vi "Main.vi"(7 "sweep rate, /min":dbl=0.2, 8 "sweep to:":dbl=4.0, 9 "sweep":T8(radio)=enum."2636a_smub") -> ()   [LabVIEW 2021] (continued)
              n2485 = property on="XY Graph" class="XYGraph (strict)"(error in=w3491, "YScale.NameLbl.Text"=w3485) -> ()  [unwired: 1 in, 2 out]
            }
            frame #1 {
              n2486 = local read "Xaxis"() -> (w3508:u16)
              n2487 = property on="Yright" class="Ring (strict)"() -> ("Value"=w3502:u16)  [unwired: 2 in, 2 out]
              n2488 = property on="Yright" class="Ring (strict)"() -> ("RingText.Text"=w3501:string)  [unwired: 2 in, 2 out]
              n2489 = property on="Xaxis" class="Ring (strict)"() -> ("RingText.Text"=w3507:string)  [unwired: 2 in, 2 out]
              n2490 = property on="Yaxis" class="Ring (strict)"() -> ("RingText.Text"=w3506:string)  [unwired: 2 in, 2 out]
              n2491 = local read "Yaxis"() -> (w3509:u16)
              n2492 = case shown="\"0\", Default" w3501 {
                tunnel: [w3514 w3521] -> w3499
                tunnel: w3502 -> [_ w3520]
                tunnel: w3503 -> [w3515 w3519]
                tunnel: [w3513 errorcluster {"status"=FALSE, "code"=0, "source"=""} ("error out")] -> _
                frame "formula" {
                  n2493 = local read "formula_variables"() -> (w3516:string[])
                  n2494 = Transpose 2D Array(2D array=w3515) -> (transposed array=w3517:dbl[][])
                  n2495 = property on="Y_right_formula" class="Str"() -> ("Value"=w3512:string)  [unwired: 2 in, 2 out]
                  n2496 = call <vilib>:"Eval Multi-Variable Array.vi"("Variables"=w3516, "X Values"=w3517, "formula"=w3512) -> ("error out"=w3513:errorcluster, "Y Values"=w3514:dbl[])  [unwired: 1 in]
                }
                frame "0", Default {
                  n2497 = Index Array(array=w3519, index (col)=w3520) -> (element=w3521:dbl[])  [unwired: 1 in]
                }
              }
              n2498 = case shown="\"formula\"" w3507 {
                tunnel: [w3532 w3537] -> w3511
                tunnel: w3508 -> [w3535 _]
                tunnel: w3503 -> [w3534 w3541]
                tunnel: [errorcluster {"status"=FALSE, "code"=0, "source"=""} ("error out") w3538] -> w3505
                tunnel: [w3532 w3537] -> w3500
                frame "0", Default {
                  n2499 = Index Array(array=w3534, index (col)=w3535) -> (element=w3532:dbl[])  [unwired: 1 in]
                }
                frame "formula" {
                  n2500 = local read "formula_variables"() -> (w3540:string[])
                  n2501 = Transpose 2D Array(2D array=w3541) -> (transposed array=w3539:dbl[][])
                  n2502 = property on="X_axis_formula" class="Str"() -> ("Value"=w3536:string)  [unwired: 2 in, 2 out]
                  n2503 = call <vilib>:"Eval Multi-Variable Array.vi"("Variables"=w3540, "X Values"=w3539, "formula"=w3536) -> ("error out"=w3538:errorcluster, "Y Values"=w3537:dbl[])  [unwired: 1 in]
                }
              }
              n2504 = case shown="\"formula\"" w3506 {
                tunnel: [w3524 w3531] -> w3510
                tunnel: w3509 -> [_ w3530]
                tunnel: w3503 -> [w3525 w3529]
                tunnel: [w3523 errorcluster {"status"=FALSE, "code"=0, "source"=""} ("error out")] -> w3504
                frame "formula" {
                  n2505 = local read "formula_variables"() -> (w3526:string[])
                  n2506 = Transpose 2D Array(2D array=w3525) -> (transposed array=w3527:dbl[][])
                  n2507 = property on="Y_left_formula" class="Str"() -> ("Value"=w3522:string)  [unwired: 2 in, 2 out]
                  n2508 = call <vilib>:"Eval Multi-Variable Array.vi"("Variables"=w3526, "X Values"=w3527, "formula"=w3522) -> ("error out"=w3523:errorcluster, "Y Values"=w3524:dbl[])  [unwired: 1 in]
                }
                frame "0", Default {
                  n2509 = Index Array(array=w3529, index (col)=w3530) -> (element=w3531:dbl[])  [unwired: 1 in]
                }
              }
              n2510 = Bundle("Y Values"=w3511, "Y Values"=w3510) -> (w3498:cluster{"Y Values":dbl[], "Y Values":dbl[]})  [unwired: 1 in]
              n2511 = Bundle("Y Values"=w3500, "Y Values"=w3499) -> (w3497:cluster{"Y Values":dbl[], "Y Values":dbl[]})  [unwired: 1 in]
              n2512 = Build Array(w3498, w3497) -> (w3496:cluster{"Y Values":dbl[], "Y Values":dbl[]}[])
              n2513 = property on="XY Graph" class="XYGraph (strict)"("Value"=w3496) -> ()  [unwired: 2 in, 2 out]
            }
            frame #2 {
              # "show if formula \nis wrong"
              n2514 = property on="Yaxis" class="Ring (strict)"() -> ("RingText.Text"=w3547:string)  [unwired: 2 in, 2 out]
              n2515 = property on="XY Graph" class="XYGraph (strict)"("Active Plot"=u32 0, "Plot.Plot Name"=w3547) -> (error out=w3548:errorcluster)  [unwired: 2 in, 1 out]
              n2516 = property on="Yright" class="Ring (strict)"() -> ("RingText.Text"=w3545:string)  [unwired: 2 in, 2 out]
              n2517 = property on="XY Graph" class="XYGraph (strict)"(error in=w3548, "Active Plot"=u32 1, "Plot.Plot Name"=w3545) -> ()  [unwired: 1 in, 2 out]
              n2518 = Unbundle By Name(w3551) -> ("status"=w3544:bool)
              n2519 = Unbundle By Name(w3550) -> ("status"=w3543:bool)
              n2520 = Unbundle By Name(w3550) -> ("status"=w3542:bool)
              n2521 = property on="status 3" class="Bool (strict)"("Value"=w3542) -> ()  [unwired: 2 in, 2 out]
              n2522 = property on="status 2" class="Bool (strict)"("Value"=w3544) -> ()  [unwired: 2 in, 2 out]
              n2523 = property on="status" class="Bool (strict)"("Value"=w3543) -> ()  [unwired: 2 in, 2 out]
            }
          }
          n2524 = stacked-sequence "set next value in the sweep" {
            tunnel: w2536 -> [w3354 _]
            tunnel: [w3354 _] -> w2535
            tunnel: w2533 -> [_ w3475]
            tunnel: w2528 -> [w3357 _]
            frame #0 {
              n2525 = local read "sweep"() -> (w3360:T8)
              n2526 = property on="Sweep Channel" class="DigNum (strict)"("Value"=w3354) -> ()  [unwired: 2 in, 2 out]
              n2527 = property on="sweep value" class="DigNum (strict)"("Value"=w3354) -> ()  [unwired: 2 in, 2 out]
              n2528 = case shown="\"AuxOut0\"" w3360 {
                tunnel: w3354 -> [w3373 w3381 w3387 w3396 w3418 _ w3420 w3443 w3467 w3470]
                tunnel: w3357 -> [_ _ _ w3394 _ _ _ _ _ _]
                frame "2400_1" {
                  # "sweep voltage on 2400 1"
                  n2529 = local read "2400 1 addr"() -> (w3375:u8)
                  n2530 = Number To Fractional String(number=w3373) -> (F-format string=w3379:string)  [unwired: 3 in]
                  n2531 = Concatenate Strings(":INIT:IMM; :SOUR:VOLT:LEV:IMM:AMPL " ("data"), w3379) -> (w3377:string)
                  n2532 = Number To Decimal String(number=w3375) -> (decimal integer string=w3374:string)  [unwired: 1 in]
                  n2533 = GPIB Write(0:w3374, 1:w3377, 2:i16 1 ("mode (0)")) -> ()  [unwired: 2 in, 2 out]
                }
                frame "2400_2" {
                  # "sweep curr on 2400 2"
                  n2534 = Number To Fractional String(number=w3381) -> (F-format string=w3386:string)  [unwired: 3 in]
                  n2535 = local read "2400 2 addr"() -> (w3383:u8)
                  n2536 = Concatenate Strings(":INIT:IMM; :SOUR:CURR:LEV:IMM:AMPL " ("data"), w3386) -> (w3384:string)
                  n2537 = Number To Decimal String(number=w3383) -> (decimal integer string=w3382:string)  [unwired: 1 in]
                  n2538 = GPIB Write(0:w3382, 1:w3384, 2:i16 1 ("mode (0)")) -> ()  [unwired: 2 in, 2 out]
                }
                frame "2400_3" {
                  # "sweep voltage on 2400 3"
                  n2539 = local read "2400 3 addr"() -> (w3389:u8)
                  n2540 = Number To Fractional String(number=w3387) -> (F-format string=w3393:string)  [unwired: 3 in]
                  n2541 = Concatenate Strings(":INIT:IMM; :SOUR:VOLT:LEV:IMM:AMPL " ("data"), w3393) -> (w3391:string)
                  n2542 = Number To Decimal String(number=w3389) -> (decimal integer string=w3388:string)  [unwired: 1 in]
                  n2543 = GPIB Write(0:w3388, 1:w3391, 2:i16 1 ("mode (0)")) -> ()  [unwired: 2 in, 2 out]
                }
                frame "2636a_smua" {
                  n2544 = case shown="False" "sweep" {
                    tunnel: w3396 -> [w3401 w3414]
                    tunnel: w3394 -> [w3398 _]
                    frame True {
                      w3399 = 30.0 ("y")
                      n2545 = Subtract(x=w3401, y=w3398) -> (x-y=w3400:dbl)
                      n2546 = Divide(x=w3400, y=w3399) -> (x/y=w3397:dbl)
                      n2547 = for {
                        N: w3399 -> [_]
                        tunnel: w3398 -> [w3407]
                        tunnel: w3397 -> [w3405]
                        i -> [w3406]
                        n2548 = Multiply(x=w3405, y=w3406) -> (x*y=w3404:dbl)
                        n2549 = local read "2614A addr"() -> (w3409:refnum<visa-resource-name>)
                        n2550 = Add(x=w3404, y=w3407) -> (x+y=w3403:dbl)
                        n2551 = call "setLevel.vi"("VISA resource name 2"=w3409, "Source"=Source."Voltage", "Channel"=Channel."a", "SourceLevel"=w3403) -> ()  [unwired: 1 in, 3 out]
                        n2552 = Wait (ms)(milliseconds to wait=u32 12) -> ()  [unwired: 1 out]
                      }
                    }
                    frame False {
                      # "sweep voltage on 2636a smua"
                      n2553 = local read "2614A addr"() -> (w3412:refnum<visa-resource-name>)
                      n2554 = call "setLevel.vi"("VISA resource name 2"=w3412, "Source"=Source."Voltage", "Channel"=Channel."a", "SourceLevel"=w3414) -> ()  [unwired: 1 in, 3 out]
                    }
                  }
                }
                frame "2636a_smub" {
                  # "sweep voltage on 2636b smua"
                  n2555 = local read "2614A addr"() -> (w3415:refnum<visa-resource-name>)
                  n2556 = call "setLevel.vi"("VISA resource name 2"=w3415, "Source"=Source."Voltage", "Channel"=Channel."b", "SourceLevel"=w3418) -> ()  [unwired: 1 in, 3 out]
                }
                frame "time_sweep", Default {
                  # "do not sweep, just time"
                }
                frame "iPS" {
                  n2557 = property on="Sweep B" class="Bool (strict)"() -> ("Value"=w3419:bool)  [unwired: 2 in, 2 out]
                  n2558 = case shown="True" w3419 {
                    tunnel: w3420 -> [_ w3421]
                    frame False {
                      # "Time as dummy B field"
                    }
                    frame True {
                      n2559 = stacked-sequence {
                        tunnel: w3421 -> [w3424 _ w3432 w3434]
                        frame #0 {
                          n2560 = local read "iPS_addr_sweep"() -> (w3423:refnum<visa-resource-name>)
                          n2561 = call "iPSset.vi"("Target Field, T"=w3424, "iPSSetCtrl"=iPSsetCtrl."Set Target Field", "VISA resource name"=w3423) -> ()  [unwired: 5 in, 4 out]
                        }
                        frame #1 {
                          n2562 = local read "iPS_addr_sweep"() -> (w3427:refnum<visa-resource-name>)
                          n2563 = property on="sweep rate, /min" class="DigNum (strict)"() -> ("Value"=w3425:dbl)  [unwired: 2 in, 2 out]
                          n2564 = call "iPSset.vi"("Field Rate, T/min"=w3425, "iPSSetCtrl"=iPSsetCtrl."Set Target Field Rate", "VISA resource name"=w3427) -> ()  [unwired: 5 in, 4 out]
                        }
                        frame #2 {
                          n2565 = Not Equal To 0?(x=w3432) -> (x != 0?=w3430:bool)
                          n2566 = local read "iPS_addr_sweep"() -> (w3433:refnum<visa-resource-name>)
                          n2567 = Select(t=iPSsetCtrl."Go to Field" ("iPSSetCtrl"), s=w3430, f=iPSsetCtrl."Go to Field" ("iPSSetCtrl")) -> (s? t:f=w3428:T16)
                          n2568 = call "iPSset.vi"("iPSSetCtrl"=w3428, "VISA resource name"=w3433) -> ()  [unwired: 6 in, 4 out]
                        }
                        frame #3 {
                          n2569 = while {
                            tunnel: w3434 -> [w3437]
                            stop <- w3440 stop-if-true
                            n2570 = property on="iPS_addr_sweep" class="VISAName"() -> ("Value"=w3436:refnum<visa-resource-name>)  [unwired: 2 in, 2 out]
                            n2571 = call "iPSread.vi"("iPSreadCtrl"=iPSreadCtrl."MagnetField", "VISA resource name"=w3436) -> ("number"=w3439:dbl)  [unwired: 6 in, 3 out]
                            n2572 = property on="Tolerance_Sweep" class="DigNum (strict)"() -> ("Value"=w3438:dbl)  [unwired: 2 in, 2 out]
                            n2573 = Subtract(x=w3439, y=w3437) -> (x-y=w3442:dbl)
                            n2574 = Absolute Value(x=w3442) -> (abs(x)=w3441:dbl)
                            n2575 = Less Or Equal?(x=w3441, y=w3438) -> (x <= y?=w3440:bool)
                          }
                        }
                      }
                    }
                  }
                }
                frame "iTC" {
                  n2576 = stacked-sequence {
                    tunnel: w3443 -> [w3445 w3452 w3457]
                    frame #0 {
                      n2577 = Decrement(x=w3445) -> (x-1=w3447:dbl)
                      n2578 = Less Or Equal To 0?(x=w3447) -> (x <= 0?=w3449:bool)
                      n2579 = Select(t=0.0, s=w3449, f=w3447) -> (s? t:f=w3446:dbl)
                      n2580 = property on="iPS_addr_sweep" class="VISAName"() -> ("Value"=w3444:refnum<visa-resource-name>)  [unwired: 2 in, 2 out]
                      n2581 = call "iTCset.vi"("Set Point"=w3446, "iTCSetCtrl"=iTCsetCtrl."Set VTI Temp", "VISA resource name"=w3444) -> ()  [unwired: 5 in, 4 out]
                    }
                    frame #1 {
                      n2582 = Less Or Equal To 0?(x=w3452) -> (x <= 0?=w3455:bool)
                      n2583 = property on="iPS_addr_sweep" class="VISAName"() -> ("Value"=w3451:refnum<visa-resource-name>)  [unwired: 2 in, 2 out]
                      n2584 = Select(t=0.0, s=w3455, f=w3452) -> (s? t:f=w3453:dbl)
                      n2585 = call "iTCset.vi"("Set Point"=w3453, "iTCSetCtrl"=iTCsetCtrl."Set Sample Temp", "VISA resource name"=w3451) -> ()  [unwired: 5 in, 4 out]
                    }
                    frame #2 {
                      n2586 = disable-structure shown="Disabled" {
                        disable-tunnel: w3457 -> [w3458 _]
                        frame Disabled {
                          n2587 = while {
                            tunnel: w3458 -> [w3461]
                            stop <- w3462 stop-if-true
                            n2588 = call "iTCread.vi"("iTCreadCtrl"=iTCreadCtrl."Sample Temp") -> ("number"=w3465:dbl, "VISA resource name"=w3459:refnum<visa-resource-name>)  [unwired: 6 in, 3 out]
                            n2589 = Subtract(x=w3465, y=w3461) -> (x-y=w3464:dbl)
                            n2590 = property on="Tolerance_Sweep" class="DigNum (strict)"() -> ("Value"=w3460:dbl)  [unwired: 2 in, 2 out]
                            n2591 = Absolute Value(x=w3464) -> (abs(x)=w3463:dbl)
                            n2592 = Less?(x=w3463, y=w3460) -> (x < y?=w3462:bool)
                          }
                        }
                        frame Enabled {
                        }
                      }
                    }
                  }
                }
                frame "2461" {
                  w3468 = u16 1 items=["Volts", "Current"] ("Function (0: Volts)")
                  n2593 = property on="2461_addr_sweep" class="VISAName"() -> ("Value"=w3469:refnum<visa-resource-name>)  [unwired: 2 in, 2 out]
                  n2594 = call <instrlib>:"Configure Source Level.vi"("Source Level (1.0)"=w3467, "Function (0: Volts)"=w3468, "VISA resource name"=w3469) -> ()  [unwired: 7 in, 2 out]
                }
                frame "AuxOut0" {
                  n2595 = property on="HandleOut" class="Clust (strict)"() -> ("Value"=w3472:T1)  [unwired: 2 in, 2 out]
                  n2596 = call "MFLIcontrol.vi"("Value"=w3470, "MFLI function"=MFLIcommand."Set AuxOut0", "handle in"=w3472) -> ()  [unwired: 4 in, 5 out]
                }
              }
              n2597 = property on="Slope" class="DigNum (strict)"() -> ("Value"=w3355:dbl)  [unwired: 2 in, 2 out]
              n2598 = property on="Offset" class="DigNum (strict)"() -> ("Value"=w3356:dbl)  [unwired: 2 in, 2 out]
              n2599 = Multiply(x=w3355, y=w3354) -> (x*y=w3358:dbl)
              n2600 = local read "sweep"() -> (w3352:T8)
              n2601 = property on="Double Sweep" class="Bool (strict)"() -> ("Value"=w3351:bool)  [unwired: 2 in, 2 out]
              n2602 = Add(x=w3356, y=w3358) -> (x+y=w3359:dbl)
              n2603 = property on="Lead Chanl" class="Enum (strict)"() -> ("Value"=w3353:T2)  [unwired: 2 in, 2 out]
              n2604 = Equal?(x=w3352, y=w3353) -> (x = y?=w3350:bool)
              n2605 = And(x=w3351, y=w3350) -> (x .and. y?=w3349:bool)
              n2606 = case shown="True" w3349 {
                tunnel: w3359 -> [_ w3361]
                frame False {
                }
                frame True {
                  n2607 = disable-structure shown="Disabled" {
                    disable-tunnel: w3361 -> [w3362 w3370]
                    frame Disabled {
                      # "sweep voltage on 2400 2"
                      n2608 = local read "2400 2 addr"() -> (w3363:u8)
                      n2609 = Number To Fractional String(number=w3362) -> (F-format string=w3364:string)  [unwired: 3 in]
                      n2610 = Concatenate Strings(":INIT:IMM; :SOUR:VOLT:LEV:IMM:AMPL " ("data"), w3364) -> (w3366:string)
                      n2611 = Number To Decimal String(number=w3363) -> (decimal integer string=w3367:string)  [unwired: 1 in]
                      n2612 = GPIB Write(0:w3367, 1:w3366, 2:i16 1 ("mode (0)")) -> ()  [unwired: 2 in, 2 out]
                    }
                    frame Enabled {
                      n2613 = property on="Slave Channel" class="Enum (strict)"() -> ("Value"=w3369:T3)  [unwired: 2 in, 2 out]
                      n2614 = local read "2614A addr"() -> (w3372:refnum<visa-resource-name>)
                      n2615 = call "setLevel.vi"("VISA resource name 2"=w3372, "Source"=Source."Voltage", "Channel"=w3369, "SourceLevel"=w3370) -> ()  [unwired: 1 in, 3 out]
                    }
                  }
                }
              }
            }
            frame #1 {
              # "calculate deliberate time delay for the next step"
              n2616 = Tick Count (ms)() -> (millisecond timer value=w3477:u32)
              n2617 = Subtract(x=w3477, y=w3475) -> (x-y=w3476:u32)
              n2618 = property on="time/point, sec" class="DigNum (strict)"() -> ("Value"=w3478:dbl)  [unwired: 2 in, 2 out]
              n2619 = Multiply(x=w3478, y=1000.0) -> (x*y=w3474:dbl)
              n2620 = Subtract(x=w3474, y=w3476) -> (x-y=w3473:dbl)
              n2621 = property on="time delay, ms" class="DigNum (strict)"("Value"=w3473) -> ()  [unwired: 2 in, 2 out]
            }
          }
          n2622 = Not(x="Continuous Sweep") -> (.not. x?=w2529:bool)
          n2623 = And(x=w2526, y=w2529) -> (x .and. y?=w2527:bool)
          n2624 = Or(x=w2527, y="Stop Sweep") -> (x .or. y?=w2525:bool)
        }
        n2625 = stacked-sequence {
          tunnel: w1361 -> [_ _ _]
          tunnel: w1360 -> [_ _ w2501]
          frame #0 {
            n2626 = property on="Linetrace or Mapping?" class="Bool (strict)"() -> ("Value"=w2463:bool)  [unwired: 2 in, 2 out]
            n2627 = case shown="False" w2463 {
              frame False {
                w2465 = T10."Enabled" ("Disabled")
                w2464 = T10."Enabled" ("Disabled")
                # "Return the buttons to Idle state"
                n2628 = property on="sweep" class="RadioBtnsControl (strict)"("DisabledEnum"=w2464) -> ()  [unwired: 2 in, 2 out]
                n2629 = property on="2182A 1 addr" class="DigNum (strict)"("DisabledEnum"=w2464) -> ()  [unwired: 2 in, 2 out]
                n2630 = property on="2182A 2 addr" class="DigNum (strict)"("DisabledEnum"=w2464) -> ()  [unwired: 2 in, 2 out]
                n2631 = property on="2182A 3 addr" class="DigNum (strict)"("DisabledEnum"=w2464) -> ()  [unwired: 2 in, 2 out]
                n2632 = property on="2182A 4 addr" class="DigNum (strict)"("DisabledEnum"=w2464) -> ()  [unwired: 2 in, 2 out]
                n2633 = property on="2400 1 addr" class="DigNum (strict)"("DisabledEnum"=w2464) -> ()  [unwired: 2 in, 2 out]
                n2634 = property on="2400 2 addr" class="DigNum (strict)"("DisabledEnum"=w2464) -> ()  [unwired: 2 in, 2 out]
                n2635 = property on="2400 3 addr" class="DigNum (strict)"("DisabledEnum"=w2464) -> ()  [unwired: 2 in, 2 out]
                n2636 = property on="2614A addr" class="VISAName"("DisabledEnum"=w2464) -> ()  [unwired: 2 in, 2 out]
                n2637 = property on="SR830 1 addr" class="DigNum (strict)"("DisabledEnum"=w2464) -> ()  [unwired: 2 in, 2 out]
                n2638 = property on="SR830 2 addr" class="DigNum (strict)"("DisabledEnum"=w2464) -> ()  [unwired: 2 in, 2 out]
                n2639 = property on="SR830 3 addr" class="DigNum (strict)"("DisabledEnum"=w2464) -> ()  [unwired: 2 in, 2 out]
                n2640 = property on="SR830 4 addr" class="DigNum (strict)"("DisabledEnum"=w2464) -> ()  [unwired: 2 in, 2 out]
                n2641 = property on="sweep to:" class="DigNum (strict)"("DisabledEnum"=w2465) -> ()  [unwired: 2 in, 2 out]
                n2642 = property on="sweep rate, /min" class="DigNum (strict)"("DisabledEnum"=w2465) -> ()  [unwired: 2 in, 2 out]
              }
              frame True {
              }
            }
            n2643 = property on="Stop Sweep" class="Bool"("DisabledEnum"=T10."Disabled and Grayed Out" ("Disabled")) -> ()  [unwired: 2 in, 2 out]
          }
          frame #1 {
            n2644 = stacked-sequence {
              frame #0 {
                n2645 = local read "sweep"() -> (w2492:T8)
                n2646 = Equal?(x=w2492, y=T17."Radio Selection 7" ("sweep")) -> (x = y?=w2490:bool)
                n2647 = case shown="True" w2490 {
                  frame False {
                  }
                  frame True {
                    n2648 = local read "iPS_addr_sweep"() -> (w2493:refnum<visa-resource-name>)
                    n2649 = call "iPSset.vi"("iPSSetCtrl"=iPSsetCtrl."Hold", "VISA resource name"=w2493) -> ()  [unwired: 6 in, 4 out]
                  }
                }
              }
              frame #1 {
                n2650 = local read "2636A smua meas v"() -> (w2499:bool)
                n2651 = local read "2636A smub meas v"() -> (w2497:bool)
                n2652 = local read "2636A smub meas i"() -> (w2496:bool)
                n2653 = local read "2636A smua meas i"() -> (w2498:bool)
                n2654 = Compound Arithmetic op=OR(w2499, w2498, w2497, w2496) -> (w2495:bool)
                n2655 = case shown="True" w2495 {
                  frame False {
                  }
                  frame True {
                    # "close session on 2636A"
                    n2656 = local read "2614A addr"() -> (w2500:refnum<visa-resource-name>)
                    n2657 = VISA Close(VISA resource name=w2500) -> ()  [unwired: 1 in, 1 out]
                  }
                }
              }
            }
            n2658 = stacked-sequence {
              frame #0 {
                n2659 = property on="MFLI1_d0" class="Bool (strict)"() -> ("Value"=w2473:bool)  [unwired: 2 in, 2 out]
                n2660 = property on="MFLI1_AuxOut0" class="Bool (strict)"() -> ("Value"=w2477:bool)  [unwired: 2 in, 2 out]
                n2661 = property on="MFLI1_d1" class="Bool (strict)"() -> ("Value"=w2472:bool)  [unwired: 2 in, 2 out]
                n2662 = property on="MFLI1_d2" class="Bool (strict)"() -> ("Value"=w2471:bool)  [unwired: 2 in, 2 out]
                n2663 = property on="MFLI1_d3" class="Bool (strict)"() -> ("Value"=w2470:bool)  [unwired: 2 in, 2 out]
                n2664 = Boolean To (0,1)(Boolean=w2472) -> (0, 1=w2468:i16)
                n2665 = Boolean To (0,1)(Boolean=w2473) -> (0, 1=w2469:i16)
                n2666 = Boolean To (0,1)(Boolean=w2477) -> (0, 1=w2474:i16)
                n2667 = Boolean To (0,1)(Boolean=w2471) -> (0, 1=w2467:i16)
                n2668 = Boolean To (0,1)(Boolean=w2470) -> (0, 1=w2466:i16)
                n2669 = Compound Arithmetic op=ADD(w2474, w2469, w2468, w2467, w2466) -> (w2475:i16)
                n2670 = Greater Than 0?(x=w2475) -> (x > 0?=w2476:bool)
                n2671 = case shown="True" w2476 {
                  frame False {
                  }
                  frame True {
                    n2672 = property on="HandleOut" class="Clust (strict)"() -> ("Value"=w2478:T1)  [unwired: 2 in, 2 out]
                    n2673 = call <instrlib>:"ziClose.vi"("Handle In"=w2478) -> ()  [unwired: 3 in, 2 out]
                  }
                }
              }
              frame #1 {
                n2674 = property on="MFLI2_d0" class="Bool (strict)"() -> ("Value"=w2488:bool)  [unwired: 2 in, 2 out]
                n2675 = property on="MFLI2_d1" class="Bool (strict)"() -> ("Value"=w2484:bool)  [unwired: 2 in, 2 out]
                n2676 = property on="MFLI2_d2" class="Bool (strict)"() -> ("Value"=w2483:bool)  [unwired: 2 in, 2 out]
                n2677 = property on="MFLI1_d3" class="Bool (strict)"() -> ("Value"=w2482:bool)  [unwired: 2 in, 2 out]
                n2678 = Boolean To (0,1)(Boolean=w2483) -> (0, 1=w2479:i16)
                n2679 = Boolean To (0,1)(Boolean=w2484) -> (0, 1=w2481:i16)
                n2680 = Boolean To (0,1)(Boolean=w2488) -> (0, 1=w2485:i16)
                n2681 = Boolean To (0,1)(Boolean=w2482) -> (0, 1=w2480:i16)
                n2682 = Compound Arithmetic op=ADD(w2485, w2481, w2480, w2479) -> (w2486:i16)
                n2683 = Greater Than 0?(x=w2486) -> (x > 0?=w2487:bool)
                n2684 = case shown="True" w2487 {
                  frame False {
                  }
                  frame True {
                    n2685 = property on="HandleOut 2" class="Clust (strict)"() -> ("Value"=w2489:T21)  [unwired: 2 in, 2 out]
                    n2686 = call <instrlib>:"ziClose.vi"("Handle In"=w2489) -> ()  [unwired: 3 in, 2 out]
                  }
                }
              }
            }
          }
          frame #2 {
            n2687 = property on="Linetrace or Mapping?" class="Bool (strict)"() -> ("Value"=w2502:bool)  [unwired: 2 in, 2 out]
            n2688 = case shown="False" w2502 {
              tunnel: w2501 -> [w2505 w2508]
              frame False {
                w2503 = T10."Enabled" ("Disabled")
                n2689 = Enqueue Element(queue=w2505, element="Idle") -> ()  [unwired: 2 in, 3 out]
                n2690 = property on="Sweep Down" class="Bool"("DisabledEnum"=w2503) -> ()  [unwired: 2 in, 2 out]
                n2691 = property on="Sweep Up" class="Bool"("DisabledEnum"=w2503) -> ()  [unwired: 2 in, 2 out]
              }
              frame True {
                n2692 = property on="Sweep Direction" class="Str"() -> ("Value"=w2506:string)  [unwired: 2 in, 2 out]
                n2693 = case shown="\"Sweep Up\"" w2506 {
                  tunnel: w2508 -> [w2509 w2516]
                  frame "Sweep Down", Default {
                    n2694 = stacked-sequence {
                      tunnel: w2509 -> [_ _ w2514]
                      frame #0 {
                        n2695 = property on="Sweep Direction" class="Str"("Value"="Sweep Up" ("Sweep Direction")) -> ()  [unwired: 2 in, 2 out]
                      }
                      frame #1 {
                        n2696 = property on="wait between sweeps(s)" class="DigNum (strict)"() -> ("Value"=w2513:u32)  [unwired: 2 in, 2 out]
                        n2697 = Multiply(x=w2513, y=u32 1000) -> (x*y=w2512:u32)
                        n2698 = Wait (ms)(milliseconds to wait=w2512) -> ()  [unwired: 1 out]
                      }
                      frame #2 {
                        n2699 = Enqueue Element(queue=w2514, element="Step to Next Value") -> ()  [unwired: 2 in, 3 out]
                      }
                    }
                  }
                  frame "Sweep Up" {
                    n2700 = stacked-sequence {
                      tunnel: w2516 -> [_ w2522]
                      frame #0 {
                        n2701 = property on="Table Index" class="DigNum (strict)"() -> ("Value"=w2519:dbl)  [unwired: 2 in, 2 out]
                        n2702 = Increment(x=w2519) -> (x+1=w2518:dbl)
                        n2703 = property on="at field" class="Bool (strict)"("Value"=FALSE ("at field")) -> ()  [unwired: 2 in, 2 out]
                        n2704 = property on="Table Index" class="DigNum (strict)"("Value"=w2518) -> ()  [unwired: 2 in, 2 out]
                        n2705 = property on="Sweep Direction" class="Str"("Value"="Sweep Down" ("Sweep Direction")) -> ()  [unwired: 2 in, 2 out]
                      }
                      frame #1 {
                        n2706 = Enqueue Element(queue=w2522, element="Step to Next Value") -> ()  [unwired: 2 in, 3 out]
                      }
                    }
                  }
                }
                n2707 = property on="Sweep Down" class="Bool"("DisabledEnum"=T10."Disabled and Grayed Out" ("Disabled")) -> ()  [unwired: 2 in, 2 out]
              }
            }
          }
        }
      }
      frame "Ramp To Limit" {
        w3552 = dbl[][] []  # emty array for data
        # "0 = SR830_1_ip\n1 = SR830_1_oop\n2 = SR830_2_ip\n3 = SR830_2_oop\n4 = SR830_3_ip\n5 = SR830_3_oop\n6 = SR830_4_ip \n7 = SR830_4_oop \n8 = SR830_5_ip \n9 = SR830_5_oop \n10= 2400_1_v \n11= 2400_1_i \n12 = 2400_2_v\n13 = 2400_2_i \n14 = 2400_3_v \n15 = 2400_3_i \n16 = 2182A_1_ch1 \n17 = 2182A_1_ch2 \n18 = 2182A_2_ch1 \n19 = 2182A_2_ch2\n20 = 2182A_3_ch1 \n21 = 2182A_3_ch2 \n22 = 2182A_4_ch1 \n23 = 2182A_4_ch2 \n24 = 2636A_smua_v \n25 = 2636A_smua_i \n26 = 2636A_smub_v \n27 = 2636A_smub_i \n28 = time\n29 = iPS_Field\n30 = iPS_Magnet_T\n31 = iPS__SH_T\n32 = iTC _sample_T\n33 = iTC _VTI_T\n34 = iTC _PT1_T\n35 = iTC _PT2_T\n36 = iTC _VTI_P\n37 = 2461_meas_v\n38= 2461_meas_i\n39= Step_Value\n40= HyperLoop_Step\n41= SuperHyper_Step"
        # "initial time in seconds\nfrom the beginning of month"
        n2708 = stacked-sequence {
          tunnel: [_ _ w4214 _ _] -> w3553
          frame #0 {
            n2709 = local read "2636A smua meas v"() -> (w3562:bool)
            n2710 = local read "2636A smub meas v"() -> (w3560:bool)
            n2711 = local read "2636A smub meas i"() -> (w3559:bool)
            n2712 = local read "2636A smua meas i"() -> (w3561:bool)
            n2713 = property on="sweep" class="RadioBtnsControl (strict)"() -> ("Value"=w3557:T8)  [unwired: 2 in, 2 out]
            n2714 = Compound Arithmetic op=OR(w3562, w3561, w3560, w3559) -> (w3558:bool)
            n2715 = case shown="\"AuxOut0\"" w3557 {
              frame "2400_1" {
                # "add label for the first column in the datafile"
                n2716 = stacked-sequence {
                  frame #0 {
                    n2717 = property on="data_caption" class="Str"("Value"="") -> ()  [unwired: 2 in, 2 out]
                    n2718 = property on="Figure_axis" class="Arr (strict)"("Value"=string[] [] ("Figure_axis_string")) -> ()  [unwired: 2 in, 2 out]
                  }
                  frame #1 {
                    w3565 = "V_sweep_2400_1" ("V_sweep")
                    n2719 = Concatenate Strings(w3565, "\t") -> (w3567:string)
                    n2720 = Build Array(w3565) -> (w3566:string[])
                    n2721 = property on="data_caption" class="Str"("Value"=w3567) -> ()  [unwired: 2 in, 2 out]
                    n2722 = property on="Figure_axis" class="Arr (strict)"("Value"=w3566) -> ()  [unwired: 2 in, 2 out]
                  }
                }
              }
              frame "2400_2" {
                n2723 = stacked-sequence {
                  frame #0 {
                    n2724 = property on="data_caption" class="Str"("Value"="") -> ()  [unwired: 2 in, 2 out]
                    n2725 = property on="Figure_axis" class="Arr (strict)"("Value"=string[] [] ("Figure_axis_string")) -> ()  [unwired: 2 in, 2 out]
                  }
                  frame #1 {
                    w3571 = "V_sweep_2400_2" ("V_sweep")
                    n2726 = Build Array(w3571) -> (w3572:string[])
                    n2727 = Concatenate Strings(w3571, "\t") -> (w3574:string)
                    n2728 = property on="Figure_axis" class="Arr (strict)"("Value"=w3572) -> ()  [unwired: 2 in, 2 out]
                    n2729 = property on="data_caption" class="Str"("Value"=w3574) -> ()  [unwired: 2 in, 2 out]
                  }
                }
              }
              frame "2400_3" {
                n2730 = stacked-sequence {
                  frame #0 {
                    n2731 = property on="data_caption" class="Str"("Value"="") -> ()  [unwired: 2 in, 2 out]
                    n2732 = property on="Figure_axis" class="Arr (strict)"("Value"=string[] [] ("Figure_axis_string")) -> ()  [unwired: 2 in, 2 out]
                  }
                  frame #1 {
                    w3577 = "V_sweep_2400_3" ("V_sweep")
                    n2733 = Concatenate Strings(w3577, "\t") -> (w3580:string)
                    n2734 = Build Array(w3577) -> (w3578:string[])
                    n2735 = property on="data_caption" class="Str"("Value"=w3580) -> ()  [unwired: 2 in, 2 out]
                    n2736 = property on="Figure_axis" class="Arr (strict)"("Value"=w3578) -> ()  [unwired: 2 in, 2 out]
                  }
                }
              }
              frame "2636a_smua" {
                n2737 = stacked-sequence {
                  frame #0 {
                    n2738 = property on="data_caption" class="Str"("Value"="") -> ()  [unwired: 2 in, 2 out]
                    n2739 = property on="Figure_axis" class="Arr (strict)"("Value"=string[] [] ("Figure_axis_string")) -> ()  [unwired: 2 in, 2 out]
                  }
                  frame #1 {
                    w3583 = "V_sweep_2636a_smua" ("V_sweep")
                    n2740 = Concatenate Strings(w3583, "\t") -> (w3586:string)
                    n2741 = Build Array(w3583) -> (w3584:string[])
                    n2742 = property on="data_caption" class="Str"("Value"=w3586) -> ()  [unwired: 2 in, 2 out]
                    n2743 = property on="Figure_axis" class="Arr (strict)"("Value"=w3584) -> ()  [unwired: 2 in, 2 out]
                  }
                }
              }
              frame "2636a_smub" {
                n2744 = stacked-sequence {
                  frame #0 {
                    n2745 = property on="data_caption" class="Str"("Value"="") -> ()  [unwired: 2 in, 2 out]
                    n2746 = property on="Figure_axis" class="Arr (strict)"("Value"=string[] [] ("Figure_axis_string")) -> ()  [unwired: 2 in, 2 out]
                  }
                  frame #1 {
                    w3589 = "V_sweep_2636a_smub" ("V_sweep")
                    n2747 = Build Array(w3589) -> (w3590:string[])
                    n2748 = Concatenate Strings(w3589, "\t") -> (w3592:string)
                    n2749 = property on="Figure_axis" class="Arr (strict)"("Value"=w3590) -> ()  [unwired: 2 in, 2 out]
                    n2750 = property on="data_caption" class="Str"("Value"=w3592) -> ()  [unwired: 2 in, 2 out]
                  }
                }
              }
              frame "time_sweep", Default {
                n2751 = stacked-sequence {
                  frame #0 {
                    n2752 = property on="data_caption" class="Str"("Value"="") -> ()  [unwired: 2 in, 2 out]
                    n2753 = property on="Figure_axis" class="Arr (strict)"("Value"=string[] [] ("Figure_axis_string")) -> ()  [unwired: 2 in, 2 out]
                  }
                  frame #1 {
                    w3595 = "time_sweep" ("V_sweep")
                    n2754 = Build Array(w3595) -> (w3596:string[])
                    n2755 = Concatenate Strings(w3595, "\t") -> (w3597:string)
                    n2756 = property on="Figure_axis" class="Arr (strict)"("Value"=w3596) -> ()  [unwired: 2 in, 2 out]
                    n2757 = property on="data_caption" class="Str"("Value"=w3597) -> ()  [unwired: 2 in, 2 out]
                  }
                }
              }
              frame "iPS" {
                n2758 = stacked-sequence {
                  frame #0 {
                    n2759 = property on="data_caption" class="Str"("Value"="") -> ()  [unwired: 2 in, 2 out]
                    n2760 = property on="Figure_axis" class="Arr (strict)"("Value"=string[] [] ("Figure_axis_string")) -> ()  [unwired: 2 in, 2 out]
                  }
                  frame #1 {
                    w3601 = "Teslatron_iPS_OutputField" ("V_sweep")
                    n2761 = Build Array(w3601) -> (w3602:string[])
                    n2762 = Concatenate Strings(w3601, "\t") -> (w3604:string)
                    n2763 = property on="Figure_axis" class="Arr (strict)"("Value"=w3602) -> ()  [unwired: 2 in, 2 out]
                    n2764 = property on="data_caption" class="Str"("Value"=w3604) -> ()  [unwired: 2 in, 2 out]
                  }
                }
              }
              frame "iTC" {
                n2765 = stacked-sequence {
                  frame #0 {
                    n2766 = property on="data_caption" class="Str"("Value"="") -> ()  [unwired: 2 in, 2 out]
                    n2767 = property on="Figure_axis" class="Arr (strict)"("Value"=string[] ["", "SR830_1_ip", "SR830_1_oop", "SR830_2_ip", "SR830_2_oop", "2461_meas_v", "2461_meas_i", "2636A_smua_v", "2636A_smua_i", "formula"] ("Figure_axis")) -> ()  [unwired: 2 in, 2 out]
                  }
                  frame #1 {
                    w3609 = "Teslatron_iTC_Temp"
                    n2768 = Build Array(w3609) -> (w3608:string[])
                    n2769 = Concatenate Strings(w3609, "\t") -> (w3607:string)
                    n2770 = property on="data_caption" class="Str"("Value"=w3607) -> ()  [unwired: 2 in, 2 out]
                    n2771 = property on="Figure_axis" class="Arr (strict)"("Value"=w3608) -> ()  [unwired: 2 in, 2 out]
                  }
                }
              }
              frame "2461" {
                n2772 = stacked-sequence {
                  frame #0 {
                    n2773 = property on="data_caption" class="Str"("Value"="") -> ()  [unwired: 2 in, 2 out]
                    n2774 = property on="Figure_axis" class="Arr (strict)"("Value"=string[] ["", "SR830_1_ip", "SR830_1_oop", "SR830_2_ip", "SR830_2_oop", "2461_meas_v", "2461_meas_i", "2636A_smua_v", "2636A_smua_i", "formula"] ("Figure_axis")) -> ()  [unwired: 2 in, 2 out]
                  }
                  frame #1 {
                    w3615 = "I_sweep_2461"
                    n2775 = Build Array(w3615) -> (w3614:string[])
                    n2776 = Concatenate Strings(w3615, "\t") -> (w3613:string)
                    n2777 = property on="data_caption" class="Str"("Value"=w3613) -> ()  [unwired: 2 in, 2 out]
                    n2778 = property on="Figure_axis" class="Arr (strict)"("Value"=w3614) -> ()  [unwired: 2 in, 2 out]
                  }
                }
              }
              frame "AuxOut0" {
                n2779 = stacked-sequence {
                  frame #0 {
                    n2780 = property on="data_caption" class="Str"("Value"="") -> ()  [unwired: 2 in, 2 out]
                    n2781 = property on="Figure_axis" class="Arr (strict)"("Value"=string[] ["", "SR830_1_ip", "SR830_1_oop", "SR830_2_ip", "SR830_2_oop", "2461_meas_v", "2461_meas_i", "2636A_smua_v", "2636A_smua_i", "formula"] ("Figure_axis")) -> ()  [unwired: 2 in, 2 out]
                  }
                  frame #1 {
                    w3621 = "V_Sweep_AuxOut0"
                    n2782 = Build Array(w3621) -> (w3620:string[])
                    n2783 = Concatenate Strings(w3621, "\t") -> (w3619:string)
                    n2784 = property on="data_caption" class="Str"("Value"=w3619) -> ()  [unwired: 2 in, 2 out]
                    n2785 = property on="Figure_axis" class="Arr (strict)"("Value"=w3620) -> ()  [unwired: 2 in, 2 out]
                  }
                }
              }
            }
            n2786 = case shown="True" w3558 {
              frame False {
              }
              frame True {
                # "opens session for 2636a system sourcemeter"
                n2787 = local read "2614A addr"() -> (w3623:refnum<visa-resource-name>)
                n2788 = VISA Open(VISA resource name=w3623) -> ()  [unwired: 4 in, 2 out]
              }
            }
          }
          frame #1 {
            # "0 = SR830_1_ip\n1 = SR830_1_oop\n2 = SR830_2_ip\n3 = SR830_2_oop\n4 = SR830_3_ip\n5 = SR830_3_oop\n6 = SR830_4_ip \n7 = SR830_4_oop \n8 = SR830_5_ip \n9 = SR830_5_oop \n10= 2400_1_v \n11= 2400_1_i \n12 = 2400_2_v\n13 = 2400_2_i \n14 = 2400_3_v \n15 = 2400_3_i \n16 = 2182A_1_ch1 \n17 = 2182A_1_ch2 \n18 = 2182A_2_ch1 \n19 = 2182A_2_ch2\n20 = 2182A_3_ch1 \n21 = 2182A_3_ch2 \n22 = 2182A_4_ch1 \n23 = 2182A_4_ch2 \n24 = 2636A_smua_v \n25 = 2636A_smua_i \n26 = 2636A_smub_v \n27 = 2636A_smub_i \n28 = time\n29 = iPS_Field\n30 = iPS_Magnet_T\n31 = iPS__SH_T\n32 = iTC _sample_T\n33 = iTC _VTI_T\n34 = iTC _PT1_T\n35 = iTC _PT2_T\n36 = iTC _VTI_P\n37 = 2461_meas_v\n38= 2461_meas_i\n39= Step_Value\n40= HyperLoop_Step\n41= SuperHyper_Step"
            # "this part constructs the first (text) line for the data file with names of all measured variables,\nalso constructs a text array contaning names of all measured variable for the \"ring\" (so parameter can be selected and plotted)"
            n2789 = stacked-sequence {
              tunnel: [w3624 _ _ _ _ _ _ _ _ _ _ _ _ _ _ _ _ _ _ _ _ _ _ _ _ _ _ _ _ _ _ _ _ _ _ _ _ _ _ _] -> _
              frame #0 {
                # "SR830 1 in phase (SR830_1_ip)"
                n2790 = local read "SR830 1 ip"() -> (w3629:bool)
                n2791 = property on="Figure_axis" class="Arr (strict)"() -> ("Value"=w3626:string[])  [unwired: 2 in, 2 out]
                n2792 = property on="data_caption" class="Str"() -> ("Value"=w3628:string)  [unwired: 2 in, 2 out]
                n2793 = case shown="True" w3629 {
                  tunnel: w3628 -> [w3631 w3637]
                  tunnel: [w3631 w3636] -> w3627
                  tunnel: w3626 -> [w3630 w3634]
                  tunnel: [w3630 w3632] -> w3625
                  frame False {
                    # "not measure SR830 1 in phase signal (SR830_1_ip)"
                  }
                  frame True {
                    w3633 = "SR830_1_ip"
                    # "measure SR830 1 in phase signal (SR830_1_ip)"
                    n2794 = local read "SR830 1 addr"() -> (w3638:u8)
                    n2795 = Number To Decimal String(number=w3638) -> (decimal integer string=w3639:string)  [unwired: 1 in]
                    n2796 = GPIB Clear(3:w3639) -> ()  [unwired: 1 in, 2 out]
                    n2797 = Build Array (concatenate)(w3634, w3633) -> (w3632:string[])
                    n2798 = Concatenate Strings(w3637, w3633, "\t") -> (w3636:string)
                  }
                }
                n2799 = property on="Figure_axis" class="Arr (strict)"("Value"=w3625) -> ()  [unwired: 2 in, 2 out]
                n2800 = property on="data_caption" class="Str"("Value"=w3627) -> (error out=w3624:errorcluster)  [unwired: 2 in, 1 out]
              }
              frame #1 {
                # "SR830 1 out of phase (SR830_1_oop)"
                n2801 = local read "SR830 1 oop"() -> (w3644:bool)
                n2802 = property on="Figure_axis" class="Arr (strict)"() -> ("Value"=w3641:string[])  [unwired: 2 in, 2 out]
                n2803 = property on="data_caption" class="Str"() -> ("Value"=w3643:string)  [unwired: 2 in, 2 out]
                n2804 = case shown="False" w3644 {
                  tunnel: w3643 -> [w3646 w3652]
                  tunnel: [w3646 w3651] -> w3642
                  tunnel: w3641 -> [w3645 w3649]
                  tunnel: [w3645 w3647] -> w3640
                  frame False {
                    # "not measure SR830 1 out of phase signal (SR830_1_oop)"
                  }
                  frame True {
                    w3648 = "SR830_1_oop"
                    # "measure SR830 1 out of phase signal (SR830_1_oop)"
                    n2805 = local read "SR830 1 addr"() -> (w3653:u8)
                    n2806 = Number To Decimal String(number=w3653) -> (decimal integer string=w3654:string)  [unwired: 1 in]
                    n2807 = GPIB Clear(3:w3654) -> ()  [unwired: 1 in, 2 out]
                    n2808 = Build Array (concatenate)(w3649, w3648) -> (w3647:string[])
                    n2809 = Concatenate Strings(w3652, w3648, "\t") -> (w3651:string)
                  }
                }
                n2810 = property on="Figure_axis" class="Arr (strict)"("Value"=w3640) -> ()  [unwired: 2 in, 2 out]
                n2811 = property on="data_caption" class="Str"("Value"=w3642) -> ()  [unwired: 2 in, 2 out]
              }
              frame #2 {
                # "SR830 2 in phase (SR830_2_ip)"
                n2812 = local read "SR830 2 ip"() -> (w3659:bool)
                n2813 = property on="Figure_axis" class="Arr (strict)"() -> ("Value"=w3656:string[])  [unwired: 2 in, 2 out]
                n2814 = property on="data_caption" class="Str"() -> ("Value"=w3658:string)  [unwired: 2 in, 2 out]
                n2815 = case shown="False" w3659 {
                  tunnel: w3658 -> [w3661 w3667]
                  tunnel: [w3661 w3666] -> w3657
                  tunnel: w3656 -> [w3660 w3664]
                  tunnel: [w3660 w3662] -> w3655
                  frame False {
                    # "not measure SR830 2 in phase signal (SR830_2_ip)"
                  }
                  frame True {
                    w3663 = "SR830_2_ip"
                    # "measure SR830 2 in phase signal (SR830_2_ip)"
                    n2816 = local read "SR830 2 addr"() -> (w3668:u8)
                    n2817 = Number To Decimal String(number=w3668) -> (decimal integer string=w3669:string)  [unwired: 1 in]
                    n2818 = GPIB Clear(3:w3669) -> ()  [unwired: 1 in, 2 out]
                    n2819 = Build Array (concatenate)(w3664, w3663) -> (w3662:string[])
                    n2820 = Concatenate Strings(w3667, w3663, "\t") -> (w3666:string)
                  }
                }
                n2821 = property on="Figure_axis" class="Arr (strict)"("Value"=w3655) -> ()  [unwired: 2 in, 2 out]
                n2822 = property on="data_caption" class="Str"("Value"=w3657) -> ()  [unwired: 2 in, 2 out]
              }
              frame #3 {
                # "SR830 2 out of phase (SR830_2_oop)"
                n2823 = local read "SR830 2 oop"() -> (w3674:bool)
                n2824 = property on="Figure_axis" class="Arr (strict)"() -> ("Value"=w3671:string[])  [unwired: 2 in, 2 out]
                n2825 = property on="data_caption" class="Str"() -> ("Value"=w3673:string)  [unwired: 2 in, 2 out]
                n2826 = case shown="False" w3674 {
                  tunnel: w3673 -> [w3676 w3682]
                  tunnel: [w3676 w3681] -> w3672
                  tunnel: w3671 -> [w3675 w3679]
                  tunnel: [w3675 w3677] -> w3670
                  frame False {
                    # "not measure SR830 2 out of phase signal (SR830_2_oop)"
                  }
                  frame True {
                    w3678 = "SR830_2_oop"
                    # "measure SR830 2 out of phase signal (SR830_2_oop)"
                    n2827 = local read "SR830 2 addr"() -> (w3683:u8)
                    n2828 = Number To Decimal String(number=w3683) -> (decimal integer string=w3684:string)  [unwired: 1 in]
                    n2829 = GPIB Clear(3:w3684) -> ()  [unwired: 1 in, 2 out]
                    n2830 = Build Array (concatenate)(w3679, w3678) -> (w3677:string[])
                    n2831 = Concatenate Strings(w3682, w3678, "\t") -> (w3681:string)
                  }
                }
                n2832 = property on="Figure_axis" class="Arr (strict)"("Value"=w3670) -> ()  [unwired: 2 in, 2 out]
                n2833 = property on="data_caption" class="Str"("Value"=w3672) -> ()  [unwired: 2 in, 2 out]
              }
              frame #4 {
                # "SR830 3 in phase (SR830_3_ip)"
                n2834 = local read "SR830 3 ip"() -> (w3689:bool)
                n2835 = property on="Figure_axis" class="Arr (strict)"() -> ("Value"=w3686:string[])  [unwired: 2 in, 2 out]
                n2836 = property on="data_caption" class="Str"() -> ("Value"=w3688:string)  [unwired: 2 in, 2 out]
                n2837 = case shown="False" w3689 {
                  tunnel: w3688 -> [w3691 w3697]
                  tunnel: [w3691 w3696] -> w3687
                  tunnel: w3686 -> [w3690 w3694]
                  tunnel: [w3690 w3692] -> w3685
                  frame False {
                    # "not measure SR830 3 in phase signal (SR830_3_ip)"
                  }
                  frame True {
                    w3693 = "SR830_3_ip"
                    # "measure SR830 3 in phase signal (SR830_3_ip)"
                    n2838 = local read "SR830 3 addr"() -> (w3698:u8)
                    n2839 = Number To Decimal String(number=w3698) -> (decimal integer string=w3699:string)  [unwired: 1 in]
                    n2840 = GPIB Clear(3:w3699) -> ()  [unwired: 1 in, 2 out]
                    n2841 = Build Array (concatenate)(w3694, w3693) -> (w3692:string[])
                    n2842 = Concatenate Strings(w3697, w3693, "\t") -> (w3696:string)
                  }
                }
                n2843 = property on="Figure_axis" class="Arr (strict)"("Value"=w3685) -> ()  [unwired: 2 in, 2 out]
                n2844 = property on="data_caption" class="Str"("Value"=w3687) -> ()  [unwired: 2 in, 2 out]
              }
              frame #5 {
                # "SR830 3 out of phase (SR830_3_oop)"
                n2845 = local read "SR830 3 oop"() -> (w3704:bool)
                n2846 = property on="Figure_axis" class="Arr (strict)"() -> ("Value"=w3701:string[])  [unwired: 2 in, 2 out]
                n2847 = property on="data_caption" class="Str"() -> ("Value"=w3703:string)  [unwired: 2 in, 2 out]
                n2848 = case shown="False" w3704 {
                  tunnel: w3703 -> [w3706 w3712]
                  tunnel: [w3706 w3711] -> w3702
                  tunnel: w3701 -> [w3705 w3709]
                  tunnel: [w3705 w3707] -> w3700
                  frame False {
                    # "not measure SR830 3 out of phase signal (SR830_3_oop)"
                  }
                  frame True {
                    w3708 = "SR830_3_oop"
                    # "measure SR830 3 out phase signal (SR830_3_oop)"
                    n2849 = local read "SR830 3 addr"() -> (w3713:u8)
                    n2850 = Number To Decimal String(number=w3713) -> (decimal integer string=w3714:string)  [unwired: 1 in]
                    n2851 = GPIB Clear(3:w3714) -> ()  [unwired: 1 in, 2 out]
                    n2852 = Build Array (concatenate)(w3709, w3708) -> (w3707:string[])
                    n2853 = Concatenate Strings(w3712, w3708, "\t") -> (w3711:string)
                  }
                }
                n2854 = property on="Figure_axis" class="Arr (strict)"("Value"=w3700) -> ()  [unwired: 2 in, 2 out]
                n2855 = property on="data_caption" class="Str"("Value"=w3702) -> ()  [unwired: 2 in, 2 out]
              }
              frame #6 {
                # "SR830 4 in phase (SR830_4_ip)"
                n2856 = local read "SR830 4 ip"() -> (w3719:bool)
                n2857 = property on="Figure_axis" class="Arr (strict)"() -> ("Value"=w3716:string[])  [unwired: 2 in, 2 out]
                n2858 = property on="data_caption" class="Str"() -> ("Value"=w3718:string)  [unwired: 2 in, 2 out]
                n2859 = case shown="False" w3719 {
                  tunnel: w3718 -> [w3721 w3727]
                  tunnel: [w3721 w3726] -> w3717
                  tunnel: w3716 -> [w3720 w3724]
                  tunnel: [w3720 w3722] -> w3715
                  frame False {
                    # "not measure SR830 4 in phase signal (SR830_4_ip)"
                  }
                  frame True {
                    w3723 = "SR830_4_ip"
                    # "measure SR830 4 in phase signal (SR830_4_ip)"
                    n2860 = local read "SR830 4 addr"() -> (w3728:u8)
                    n2861 = Number To Decimal String(number=w3728) -> (decimal integer string=w3729:string)  [unwired: 1 in]
                    n2862 = GPIB Clear(3:w3729) -> ()  [unwired: 1 in, 2 out]
                    n2863 = Build Array (concatenate)(w3724, w3723) -> (w3722:string[])
                    n2864 = Concatenate Strings(w3727, w3723, "\t") -> (w3726:string)
                  }
                }
                n2865 = property on="Figure_axis" class="Arr (strict)"("Value"=w3715) -> ()  [unwired: 2 in, 2 out]
                n2866 = property on="data_caption" class="Str"("Value"=w3717) -> ()  [unwired: 2 in, 2 out]
              }
              frame #7 {
                # "SR830 4 out of phase (SR830_4_oop)"
                n2867 = local read "SR830 4 oop"() -> (w3734:bool)
                n2868 = property on="Figure_axis" class="Arr (strict)"() -> ("Value"=w3731:string[])  [unwired: 2 in, 2 out]
                n2869 = property on="data_caption" class="Str"() -> ("Value"=w3733:string)  [unwired: 2 in, 2 out]
                n2870 = case shown="False" w3734 {
                  tunnel: w3733 -> [w3736 w3742]
                  tunnel: [w3736 w3741] -> w3732
                  tunnel: w3731 -> [w3735 w3739]
                  tunnel: [w3735 w3737] -> w3730
                  frame False {
                    # "not measure SR830 4 out of phase signal (SR830_4_oop)"
                  }
                  frame True {
                    w3738 = "SR830_4_oop"
                    # "measure SR830 4 out of phase signal (SR830_4_oop)"
                    n2871 = local read "SR830 4 addr"() -> (w3743:u8)
                    n2872 = Number To Decimal String(number=w3743) -> (decimal integer string=w3744:string)  [unwired: 1 in]
                    n2873 = GPIB Clear(3:w3744) -> ()  [unwired: 1 in, 2 out]
                    n2874 = Build Array (concatenate)(w3739, w3738) -> (w3737:string[])
                    n2875 = Concatenate Strings(w3742, w3738, "\t") -> (w3741:string)
                  }
                }
                n2876 = property on="Figure_axis" class="Arr (strict)"("Value"=w3730) -> ()  [unwired: 2 in, 2 out]
                n2877 = property on="data_caption" class="Str"("Value"=w3732) -> ()  [unwired: 2 in, 2 out]
              }
              frame #8 {
                # "SR830 5 in phase (SR830_5_ip)"
                n2878 = local read "SR830 5 ip"() -> (w3749:bool)
                n2879 = property on="Figure_axis" class="Arr (strict)"() -> ("Value"=w3746:string[])  [unwired: 2 in, 2 out]
                n2880 = property on="data_caption" class="Str"() -> ("Value"=w3748:string)  [unwired: 2 in, 2 out]
                n2881 = case shown="True" w3749 {
                  tunnel: w3748 -> [w3751 w3757]
                  tunnel: [w3751 w3756] -> w3747
                  tunnel: w3746 -> [w3750 w3754]
                  tunnel: [w3750 w3752] -> w3745
                  frame False {
                    # "not measure SR830 5 in phase signal (SR830_5_ip)"
                  }
                  frame True {
                    w3753 = "SR830_5_ip"
                    # "measure SR830 5 in phase signal (SR830_5_ip)"
                    n2882 = local read "SR830 5 addr"() -> (w3758:u8)
                    n2883 = Number To Decimal String(number=w3758) -> (decimal integer string=w3759:string)  [unwired: 1 in]
                    n2884 = GPIB Clear(3:w3759) -> ()  [unwired: 1 in, 2 out]
                    n2885 = Build Array (concatenate)(w3754, w3753) -> (w3752:string[])
                    n2886 = Concatenate Strings(w3757, w3753, "\t") -> (w3756:string)
                  }
                }
                n2887 = property on="Figure_axis" class="Arr (strict)"("Value"=w3745) -> ()  [unwired: 2 in, 2 out]
                n2888 = property on="data_caption" class="Str"("Value"=w3747) -> ()  [unwired: 2 in, 2 out]
              }
              frame #9 {
                # "SR830 5 out of phase (SR830_5_oop)"
                n2889 = local read "SR830 5 oop"() -> (w3764:bool)
                n2890 = property on="Figure_axis" class="Arr (strict)"() -> ("Value"=w3761:string[])  [unwired: 2 in, 2 out]
                n2891 = property on="data_caption" class="Str"() -> ("Value"=w3763:string)  [unwired: 2 in, 2 out]
                n2892 = case shown="True" w3764 {
                  tunnel: w3763 -> [w3766 w3772]
                  tunnel: [w3766 w3771] -> w3762
                  tunnel: w3761 -> [w3765 w3769]
                  tunnel: [w3765 w3767] -> w3760
                  frame False {
                    # "not measure SR830 5 out of phase signal (SR830_5_oop)"
                  }
                  frame True {
                    w3768 = "SR830_4_oop"
                    # "measure SR830 5 out of phase signal (SR830_5_oop)"
                    n2893 = local read "SR830 5 addr"() -> (w3773:u8)
                    n2894 = Number To Decimal String(number=w3773) -> (decimal integer string=w3774:string)  [unwired: 1 in]
                    n2895 = GPIB Clear(3:w3774) -> ()  [unwired: 1 in, 2 out]
                    n2896 = Build Array (concatenate)(w3769, w3768) -> (w3767:string[])
                    n2897 = Concatenate Strings(w3772, w3768, "\t") -> (w3771:string)
                  }
                }
                n2898 = property on="Figure_axis" class="Arr (strict)"("Value"=w3760) -> ()  [unwired: 2 in, 2 out]
                n2899 = property on="data_caption" class="Str"("Value"=w3762) -> ()  [unwired: 2 in, 2 out]
              }
              frame #10 {
                # "2400 1 voltage measure (2400_1_v)"
                n2900 = local read "2400 1 meas v"() -> (w3779:bool)
                n2901 = property on="Figure_axis" class="Arr (strict)"() -> ("Value"=w3776:string[])  [unwired: 2 in, 2 out]
                n2902 = property on="data_caption" class="Str"() -> ("Value"=w3778:string)  [unwired: 2 in, 2 out]
                n2903 = case shown="False" w3779 {
                  tunnel: w3778 -> [w3781 w3787]
                  tunnel: [w3781 w3786] -> w3777
                  tunnel: w3776 -> [w3780 w3784]
                  tunnel: [w3780 w3782] -> w3775
                  frame False {
                    # "not measure 2400 1 voltage (2400_1_v)"
                  }
                  frame True {
                    w3783 = "2400_1_v"
                    # "measure 2400 1 voltage (2400_1_v)"
                    n2904 = local read "2400 1 addr"() -> (w3788:u8)
                    n2905 = Number To Decimal String(number=w3788) -> (decimal integer string=w3789:string)  [unwired: 1 in]
                    n2906 = GPIB Clear(3:w3789) -> ()  [unwired: 1 in, 2 out]
                    n2907 = Build Array (concatenate)(w3784, w3783) -> (w3782:string[])
